vi "control plot.vi"(8 "Coords":T1, 11 "Plot: Argan 2":refnum<vi>) -> ()   [LabVIEW 2010]
uses:
  <vilib>/Utility/miscctls.llb/LVPoint32TypeDef.ctl
panel:
  out "Plot: Argan":cluster{dbl[], dbl[]}[](graph)
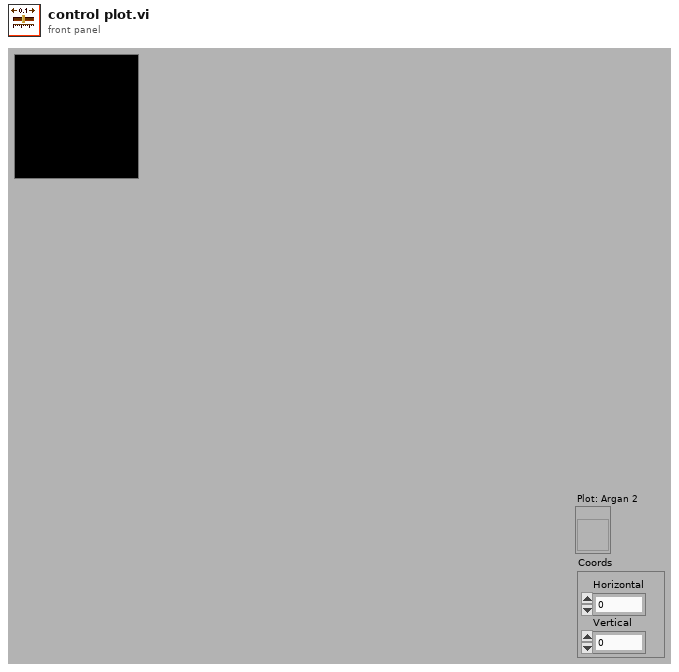
[diagram p1: front panel]
types:
  T1 = typedef "LVPoint32TypeDef.ctl" = cluster{"Horizontal":i32, "Vertical":i32}
  T2 = cluster{"Name":string, "Color":u32, "Style":u8, "Point Style":u8, "Name Visible":bool, "Allow Drag":bool, "Annotation Mode":u32, "Plot":i32, "Index":i32, "Position":cluster{"X":dbl, "Y":dbl}, "X Scale":u32, "Y Scale":u32, "Show Arrow":bool, "Lock Name":bool, "Plot Area":i32, "Label Offset":cluster{"X":dbl, "Y":dbl}}
  T3 = typedef "LVBoundsTypeDef.ctl" = cluster{"Width":u32, "Height":u32}
  T4 = typedef "LVPositionTypeDef.ctl" = cluster{"Left":i32, "Top":i32}
  T5 = cluster{"Name":string, "Color":u32, "Style":u8, "Point Style":u8, "Name Visible":bool, "Allow Drag":bool, "Annotation Mode":u32, "Plot":i32, "Index":i32, "Position":cluster{"X":dbl, "Y":dbl}, "X Scale":u32, "Y Scale":u32, "Show Arrow":bool, "Lock Name":bool, "Plot Area":i32, "Label Offset":cluster{"X":dbl, "Y":dbl}}[]
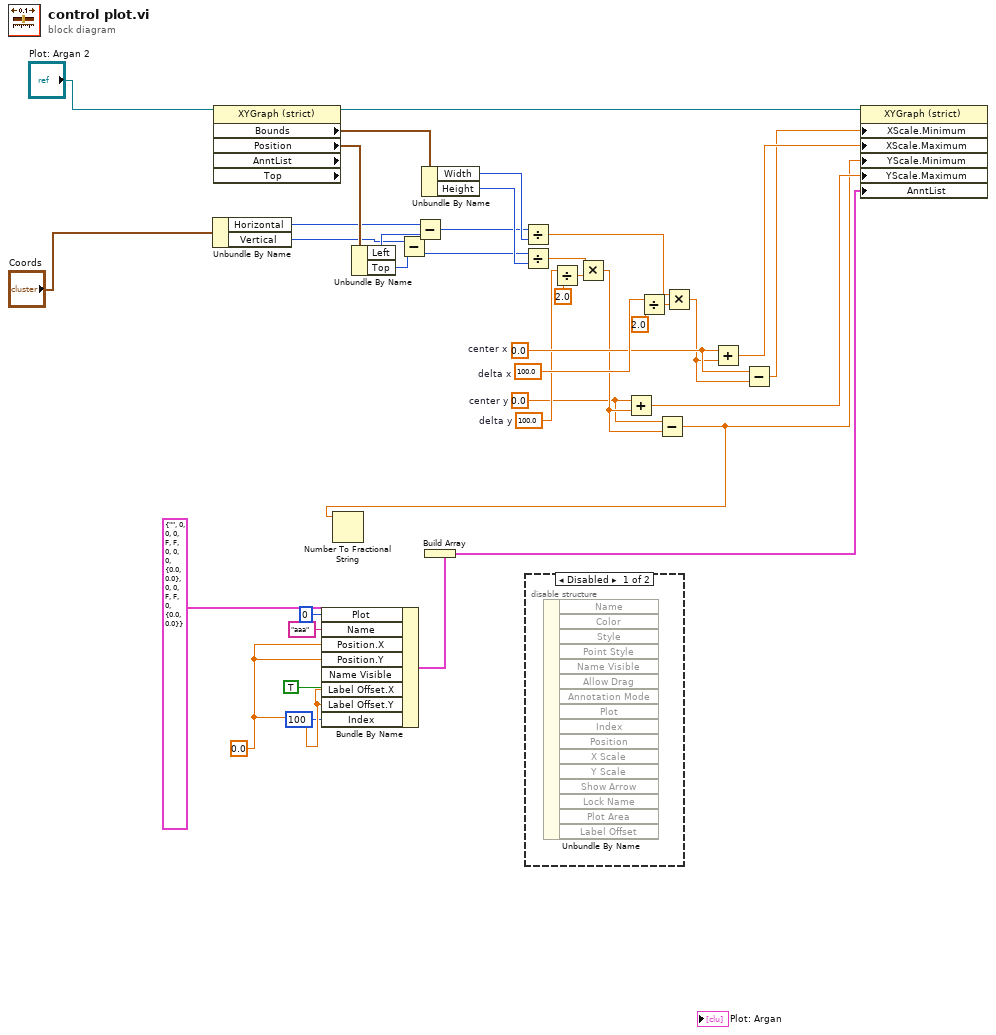
[diagram p0: block diagram]
diagram:
  w5 = 0.0 ("Position.X")
  w19 = 100.0  # delta y
  w17 = 0.0  # center y
  w28 = 100.0  # delta x
  w24 = 0.0  # center x
  n1 = Unbundle By Name("Coords") -> ("Horizontal"=w36:i32, "Vertical"=w34:i32)
  n2 = property on="Property Node" class="XYGraph (strict)" props=["Bounds", "Position", "AnntList", "Top"](reference="Plot: Argan 2") -> (reference out=w32:refnum<vi>, "Bounds"=w31:T3, "Position"=w37:T4)  [unwired: 1 in, 3 out]
  n3 = Bundle By Name(cluster=T2 {"Name"="", "Color"=0, "Style"=0, "Point Style"=0, "Name Visible"=FALSE, "Allow Drag"=FALSE, "Annotation Mode"=0, "Plot"=0, "Index"=0, "Position"={"X"=0.0, "Y"=0.0}, "X Scale"=0, "Y Scale"=0, "Show Arrow"=FALSE, "Lock Name"=FALSE, "Plot Area"=0, "Label Offset"={"X"=0.0, "Y"=0.0}}, "Plot"=0, "Name"="aaa", "Position.X"=w5, "Position.Y"=w5, "Name Visible"=TRUE, "Label Offset.X"=w5, "Label Offset.Y"=w5, "Index"=100) -> (w11:T2)
  n4 = Unbundle By Name(w37) -> ("Left"=w35:i32, "Top"=w33:i32)
  n5 = Subtract(x=w34, y=w33) -> (x-y=w8:i32)
  n6 = Subtract(x=w36, y=w35) -> (x-y=w9:i32)
  n7 = Unbundle By Name(w31) -> ("Width"=w30:u32, "Height"=w29:u32)
  n8 = Build Array(w11) -> (w10:T5)
  n9 = Divide(x=w9, y=w30) -> (x/y=w25:dbl)
  n10 = Divide(x=w8, y=w29) -> (x/y=w20:dbl)
  n11 = disable-structure shown="Disabled" {
    frame Disabled {
      n12 = Unbundle By Name() -> ()  [unwired: 1 in, 16 out]
    }
    frame Enabled {
    }
  }
  n13 = Divide(x=w19, y=2.0) -> (x/y=w21:dbl)
  n14 = Multiply(x=w20, y=w21) -> (x*y=w18:dbl)
  n15 = Add(x=w17, y=w18) -> (x+y=w14:dbl)
  n16 = Divide(x=w28, y=2.0) -> (x/y=w26:dbl)
  n17 = Subtract(x=w17, y=w18) -> (x-y=w12:dbl)
  n18 = Number To Fractional String(number=w12) -> ()  [unwired: 3 in, 1 out]
  n19 = Multiply(x=w25, y=w26) -> (x*y=w23:dbl)
  n20 = Add(x=w24, y=w23) -> (x+y=w16:dbl)
  n21 = Subtract(x=w24, y=w23) -> (x-y=w15:dbl)
  n22 = property on="Property Node" class="XYGraph (strict)"(reference=w32, "XScale.Minimum"=w15, "XScale.Maximum"=w16, "YScale.Minimum"=w12, "YScale.Maximum"=w14, "AnntList"=w10) -> ()  [unwired: 1 in, 2 out]
